vi "RSZVB Save Segment.vi"(8 "error in (no error)":errorcluster {"code" format="%.0x"}, 9 "File Name":string, 10 "Channel (1)":i32=1, 11 "VISA session":refnum<visa-resource-name>) -> (0 "error out":errorcluster {"code" format="%.0x"}, 3 "dup VISA session":refnum<visa-resource-name>)   [LabVIEW 2011]
doc: "This VI saves the sweep segment definition of a specified channel to a sweep segment file.\n\nRemote-control command(s):\nMMEMory:STORe:SEGMent <Ch>, '<file_name>'"
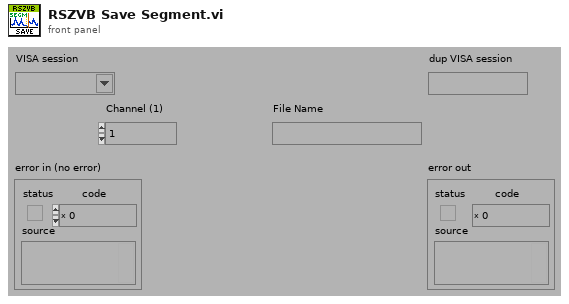
[diagram p1: front panel]
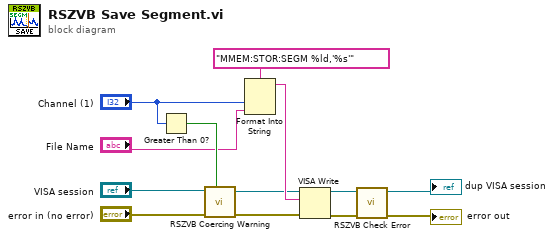
[diagram p0: block diagram]
diagram:
  n1 = Greater Than 0?(x="Channel (1)") -> (x > 0?=w10:bool)
  n2 = call "RSZVB Coercing Warning.vi"("In Range?"=w10, "error in (no error)"="error in (no error)", "VISA session"="VISA session") -> ("error out"=w7:errorcluster, "dup VISA session"=w2:refnum<visa-resource-name>)  [unwired: 7 in]
  n3 = Format Into String(format string="MMEM:STOR:SEGM %ld,'%s'", "Channel (1)", "File Name") -> (resulting string=w4:string)  [unwired: 2 in, 1 out]
  n4 = VISA Write(VISA resource name=w2, write buffer=w4, error in (no error)=w7) -> (VISA resource name out=w12:refnum<visa-resource-name>, error out=w13:errorcluster)  [unwired: 1 out]
  n5 = call "RSZVB Check Error.vi"("error in (no error)"=w13, "VISA session"=w12) -> ("error out"=→"error out":errorcluster, "dup VISA session"=→"dup VISA session":refnum<visa-resource-name>)  [unwired: 8 in]
